vi "berekeningdutycycle.vi"(11 "Graden":dbl) -> (3 "Numeric":dbl)   [LabVIEW 2014]
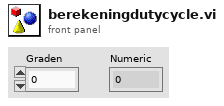
[diagram p1: front panel]
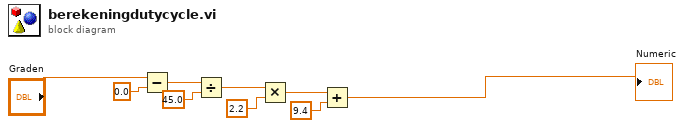
[diagram p0: block diagram]
diagram:
  n1 = Subtract(x="Graden", y=0.0) -> (x-y=w4:dbl)
  n2 = Divide(x=w4, y=45.0) -> (x/y=w5:dbl)
  n3 = Multiply(x=w5, y=2.2) -> (x*y=w6:dbl)
  n4 = Add(x=w6, y=9.4) -> (x+y=→"Numeric":dbl)
